vi "GetPositionDegreesPosition.vi"(0 "StepMotor in":refnum<class "StepMotor.lvclass">, 2 "Редукция":dbl, 3 "Разрешение энкодера":dbl, 5 "error in (no error)":errorcluster) -> (14 "StepMotor out":refnum<class "StepMotor.lvclass">, 16 "Значение":dbl, 17 "+360 -360":bool, 18 "+ 0 -":bool, 19 "error out":errorcluster)   [LabVIEW 2010, in "StepMotor.lvclass"]
uses:
  StepMotor.lvclass
panel:
  out "BadValue":bool
  out "RawValue":dbl
  out "МножПриведШкалы360":dbl
  out "КолИмпулОборот":dbl
  out "Текущая позиция":dbl
  out "Предыдущая позиция":dbl
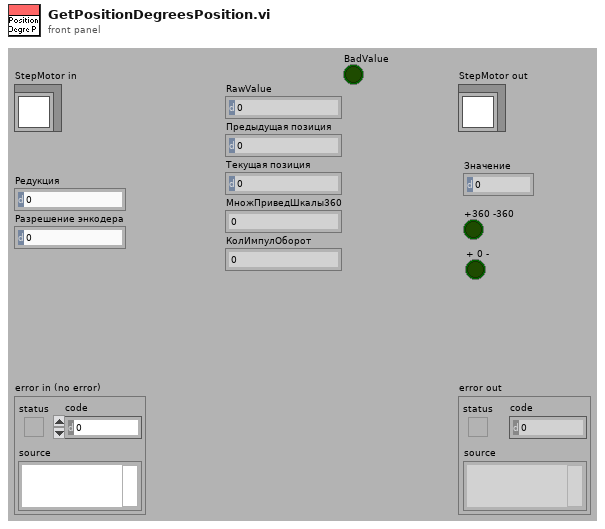
[diagram p1: front panel]
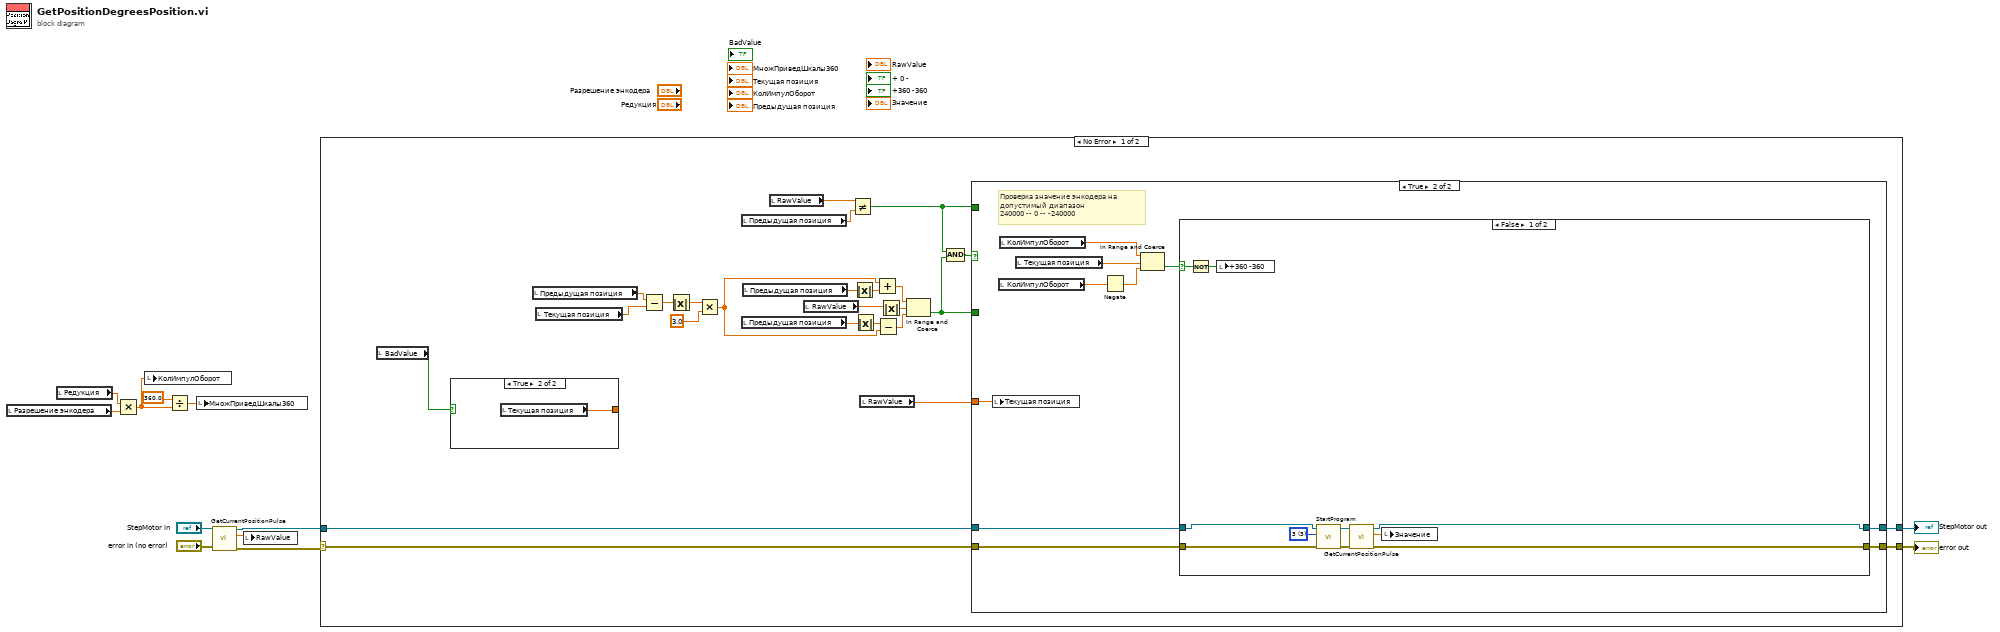
[diagram p0: block diagram]
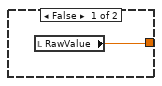
[diagram p2: hidden frame]
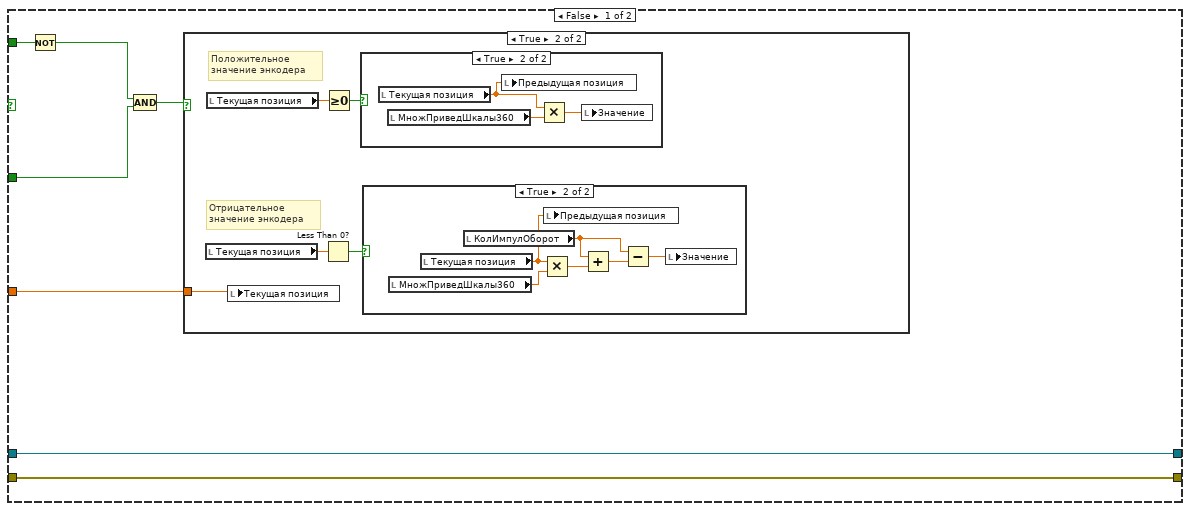
[diagram p3: hidden frame]
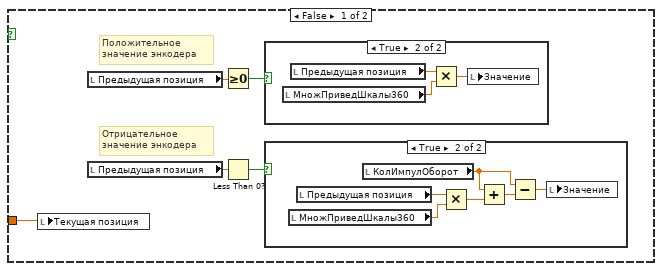
[diagram p4: hidden frame]
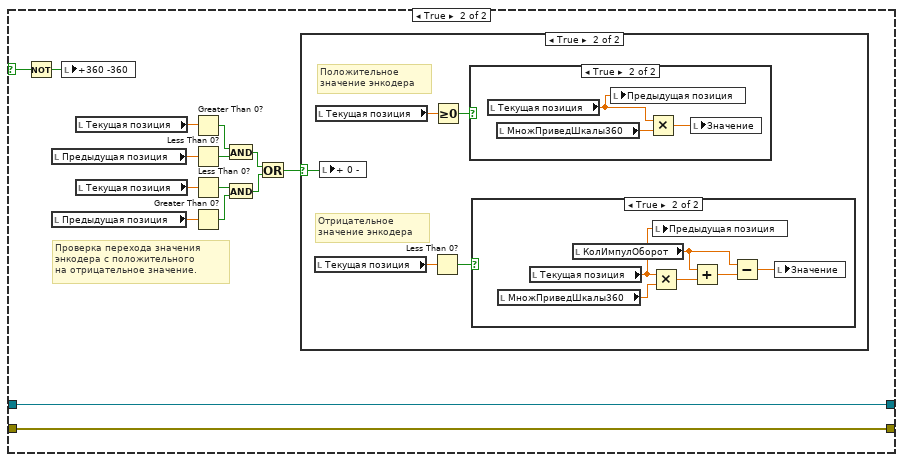
[diagram p9: hidden frame]
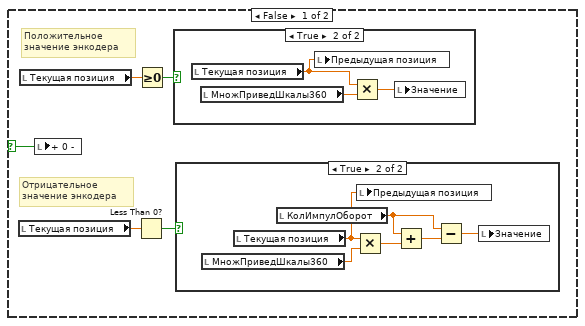
[diagram p10: hidden frame]
diagram:
  n1 = local read "Разрешение энкодера"() -> (w7:dbl)
  n2 = local read "Редукция"() -> (w6:dbl)
  n3 = Multiply(x=w6, y=w7) -> (x*y=w9:dbl)
  n4 = local write "КолИмпулОборот"(w9) -> ()
  n5 = Divide(x=360.0, y=w9) -> (x/y=w10:dbl)
  n6 = local write "МножПриведШкалы360"(w10) -> ()
  n7 = call-dynamic "GetCurrentPositionPulse.vi"("error in (no error)"="error in (no error)", "StepMotor in"="StepMotor in") -> ("error out"=w1:errorcluster, "Текущая позиция"=w5:dbl, "StepMotor out"=w2:refnum<class "StepMotor.lvclass">)  [unwired: 7 in]
  n8 = local write "RawValue"(w5) -> ()
  n9 = case shown="No Error" w1 {
    selector: w1 -> [w18 w138]
    tunnel: w2 -> [w19 w139]
    tunnel: [w37 w139] -> w11
    tunnel: [w36 w138] -> w12
    frame No Error {
      n10 = local read "BadValue"() -> (w16:bool)
      n11 = case shown="True" w16 {
        tunnel: [w38 w39] -> _
        frame False {
          n12 = local read "RawValue"() -> (w38:dbl)
        }
        frame True {
          n13 = local read "Текущая позиция"() -> (w39:dbl)
        }
      }
      n14 = local read "Предыдущая позиция"() -> (w24:dbl)
      n15 = local read "Текущая позиция"() -> (w13:dbl)
      n16 = Subtract(x=w24, y=w13) -> (x-y=w23:dbl)
      n17 = Absolute Value(x=w23) -> (abs(x)=w21:dbl)
      n18 = Multiply(x=w21, y=3.0) -> (x*y=w22:dbl)
      n19 = local read "Предыдущая позиция"() -> (w35:dbl)
      n20 = local read "Предыдущая позиция"() -> (w28:dbl)
      n21 = local read "Предыдущая позиция"() -> (w25:dbl)
      n22 = local read "RawValue"() -> (w15:dbl)
      n23 = local read "RawValue"() -> (w17:dbl)
      n24 = Not Equal?(x=w15, y=w35) -> (x != y?=w32:bool)
      n25 = Absolute Value(x=w25) -> (abs(x)=w29:dbl)
      n26 = Absolute Value(x=w28) -> (abs(x)=w27:dbl)
      n27 = local read "RawValue"() -> (w14:dbl)
      n28 = Add(x=w22, y=w29) -> (x+y=w30:dbl)
      n29 = Subtract(x=w27, y=w22) -> (x-y=w26:dbl)
      n30 = Absolute Value(x=w17) -> (abs(x)=w31:dbl)
      n31 = In Range and Coerce(upper limit=w30, x=w31, lower limit=w26) -> (In Range?=w33:bool)  [unwired: 1 out]
      n32 = Compound Arithmetic op=AND(w32, w33) -> (w34:bool)
      n33 = case shown="True" w34 {
        tunnel: w33 -> [w41 _]
        tunnel: w32 -> [w44 _]
        tunnel: w19 -> [w46 w84]
        tunnel: w18 -> [w45 w83]
        tunnel: [w46 w82] -> w37
        tunnel: [w45 w81] -> w36
        tunnel: w14 -> [w40 w75]
        frame False {
          n34 = Not(x=w44) -> (.not. x?=w43:bool)
          n35 = Compound Arithmetic op=AND(w43, w41) -> (w42:bool)
          n36 = case shown="True" w42 {
            tunnel: w40 -> [w47 w61]
            frame False {
              # "Отрицательное \nзначение энкодера"
              # "Положительное \nзначение энкодера"
              n37 = local write "Текущая позиция"(w47) -> ()
              n38 = local read "Предыдущая позиция"() -> (w49:dbl)
              n39 = local read "Предыдущая позиция"() -> (w48:dbl)
              n40 = Greater Or Equal To 0?(x=w49) -> (x >= 0?=w51:bool)
              n41 = Less Than 0?(x=w48) -> (x < 0?=w50:bool)
              n42 = case shown="True" w51 {
                frame False {
                }
                frame True {
                  n43 = local read "МножПриведШкалы360"() -> (w60:dbl)
                  n44 = local read "Предыдущая позиция"() -> (w58:dbl)
                  n45 = Multiply(x=w58, y=w60) -> (x*y=w59:dbl)
                  n46 = local write "Значение"(w59) -> ()
                }
              }
              n47 = case shown="True" w50 {
                frame False {
                }
                frame True {
                  n48 = local read "МножПриведШкалы360"() -> (w57:dbl)
                  n49 = local read "Предыдущая позиция"() -> (w56:dbl)
                  n50 = local read "КолИмпулОборот"() -> (w54:dbl)
                  n51 = Multiply(x=w56, y=w57) -> (x*y=w55:dbl)
                  n52 = Add(x=w54, y=w55) -> (x+y=w53:dbl)
                  n53 = Subtract(x=w54, y=w53) -> (x-y=w52:dbl)
                  n54 = local write "Значение"(w52) -> ()
                }
              }
            }
            frame True {
              # "Отрицательное \nзначение энкодера"
              # "Положительное \nзначение энкодера"
              n55 = local read "Текущая позиция"() -> (w65:dbl)
              n56 = local read "Текущая позиция"() -> (w64:dbl)
              n57 = local write "Текущая позиция"(w61) -> ()
              n58 = Less Than 0?(x=w65) -> (x < 0?=w62:bool)
              n59 = Greater Or Equal To 0?(x=w64) -> (x >= 0?=w63:bool)
              n60 = case shown="True" w63 {
                frame False {
                }
                frame True {
                  n61 = local read "Текущая позиция"() -> (w72:dbl)
                  n62 = local read "МножПриведШкалы360"() -> (w74:dbl)
                  n63 = local write "Предыдущая позиция"(w72) -> ()
                  n64 = Multiply(x=w72, y=w74) -> (x*y=w73:dbl)
                  n65 = local write "Значение"(w73) -> ()
                }
              }
              n66 = case shown="True" w62 {
                frame False {
                }
                frame True {
                  n67 = local read "МножПриведШкалы360"() -> (w71:dbl)
                  n68 = local read "Текущая позиция"() -> (w70:dbl)
                  n69 = local read "КолИмпулОборот"() -> (w68:dbl)
                  n70 = Multiply(x=w70, y=w71) -> (x*y=w69:dbl)
                  n71 = local write "Предыдущая позиция"(w70) -> ()
                  n72 = Add(x=w68, y=w69) -> (x+y=w67:dbl)
                  n73 = Subtract(x=w68, y=w67) -> (x-y=w66:dbl)
                  n74 = local write "Значение"(w66) -> ()
                }
              }
            }
          }
        }
        frame True {
          # "Проверка значение энкодера на\nдопустимый диапазон \n240000 -- 0 -- -240000"
          n75 = local write "Текущая позиция"(w75) -> ()
          n76 = local read "КолИмпулОборот"() -> (w77:dbl)
          n77 = local read "КолИмпулОборот"() -> (w78:dbl)
          n78 = local read "Текущая позиция"() -> (w76:dbl)
          n79 = Negate(x=w77) -> (-x=w80:dbl)
          n80 = In Range and Coerce(upper limit=w78, x=w76, lower limit=w80) -> (In Range?=w79:bool)  [unwired: 1 out]
          n81 = case shown="False" w79 {
            selector: w79 -> [w91 w95]
            tunnel: w84 -> [w88 w98]
            tunnel: w83 -> [w87 w97]
            tunnel: [w93 w98] -> w82
            tunnel: [w92 w97] -> w81
            frame False {
              w94 = u16 3 items=["0", "1", "2", "3", "4", "5", "6", "7"] ("Номер банка программ")
              n82 = Not(x=w91) -> (.not. x?=w90:bool)
              n83 = local write "+360 -360"(w90) -> ()
              n84 = call-dynamic "StartProgram.vi"("error in (no error)"=w87, "Номер банка программ"=w94, "StepMotor in"=w88) -> ("error out"=w85:errorcluster, "StepMotor out"=w86:refnum<class "StepMotor.lvclass">)  [unwired: 7 in]
              n85 = call-dynamic "GetCurrentPositionPulse.vi"("error in (no error)"=w85, "StepMotor in"=w86) -> ("error out"=w92:errorcluster, "Текущая позиция"=w89:dbl, "StepMotor out"=w93:refnum<class "StepMotor.lvclass">)  [unwired: 7 in]
              n86 = local write "Значение"(w89) -> ()
            }
            frame True {
              # "Проверка перехода значения \nэнкодера с положительного\nна отрицательное значение."
              n87 = Not(x=w95) -> (.not. x?=w96:bool)
              n88 = local read "Предыдущая позиция"() -> (w100:dbl)
              n89 = local read "Предыдущая позиция"() -> (w99:dbl)
              n90 = local write "+360 -360"(w96) -> ()
              n91 = local read "Текущая позиция"() -> (w102:dbl)
              n92 = local read "Текущая позиция"() -> (w101:dbl)
              n93 = Greater Than 0?(x=w102) -> (x > 0?=w105:bool)
              n94 = Less Than 0?(x=w100) -> (x < 0?=w106:bool)
              n95 = Less Than 0?(x=w101) -> (x < 0?=w104:bool)
              n96 = Greater Than 0?(x=w99) -> (x > 0?=w103:bool)
              n97 = And(x=w105, y=w106) -> (x .and. y?=w107:bool)
              n98 = And(x=w104, y=w103) -> (x .and. y?=w108:bool)
              n99 = Or(x=w107, y=w108) -> (x .or. y?=w109:bool)
              n100 = case shown="True" w109 {
                selector: w109 -> [w110 w124]
                frame False {
                  # "Отрицательное \nзначение энкодера"
                  # "Положительное \nзначение энкодера"
                  n101 = local read "Текущая позиция"() -> (w114:dbl)
                  n102 = local read "Текущая позиция"() -> (w113:dbl)
                  n103 = local write "+ 0 -"(w110) -> ()
                  n104 = Less Than 0?(x=w114) -> (x < 0?=w111:bool)
                  n105 = Greater Or Equal To 0?(x=w113) -> (x >= 0?=w112:bool)
                  n106 = case shown="True" w112 {
                    frame False {
                    }
                    frame True {
                      n107 = local read "Текущая позиция"() -> (w121:dbl)
                      n108 = local read "МножПриведШкалы360"() -> (w123:dbl)
                      n109 = local write "Предыдущая позиция"(w121) -> ()
                      n110 = Multiply(x=w121, y=w123) -> (x*y=w122:dbl)
                      n111 = local write "Значение"(w122) -> ()
                    }
                  }
                  n112 = case shown="True" w111 {
                    frame False {
                    }
                    frame True {
                      n113 = local read "МножПриведШкалы360"() -> (w120:dbl)
                      n114 = local read "Текущая позиция"() -> (w119:dbl)
                      n115 = local read "КолИмпулОборот"() -> (w117:dbl)
                      n116 = Multiply(x=w119, y=w120) -> (x*y=w118:dbl)
                      n117 = local write "Предыдущая позиция"(w119) -> ()
                      n118 = Add(x=w117, y=w118) -> (x+y=w116:dbl)
                      n119 = Subtract(x=w117, y=w116) -> (x-y=w115:dbl)
                      n120 = local write "Значение"(w115) -> ()
                    }
                  }
                }
                frame True {
                  # "Отрицательное \nзначение энкодера"
                  # "Положительное \nзначение энкодера"
                  n121 = local read "Текущая позиция"() -> (w128:dbl)
                  n122 = local read "Текущая позиция"() -> (w127:dbl)
                  n123 = local write "+ 0 -"(w124) -> ()
                  n124 = Less Than 0?(x=w128) -> (x < 0?=w125:bool)
                  n125 = Greater Or Equal To 0?(x=w127) -> (x >= 0?=w126:bool)
                  n126 = case shown="True" w126 {
                    frame False {
                    }
                    frame True {
                      n127 = local read "Текущая позиция"() -> (w135:dbl)
                      n128 = local read "МножПриведШкалы360"() -> (w137:dbl)
                      n129 = local write "Предыдущая позиция"(w135) -> ()
                      n130 = Multiply(x=w135, y=w137) -> (x*y=w136:dbl)
                      n131 = local write "Значение"(w136) -> ()
                    }
                  }
                  n132 = case shown="True" w125 {
                    frame False {
                    }
                    frame True {
                      n133 = local read "МножПриведШкалы360"() -> (w134:dbl)
                      n134 = local read "Текущая позиция"() -> (w133:dbl)
                      n135 = local read "КолИмпулОборот"() -> (w131:dbl)
                      n136 = Multiply(x=w133, y=w134) -> (x*y=w132:dbl)
                      n137 = local write "Предыдущая позиция"(w133) -> ()
                      n138 = Add(x=w131, y=w132) -> (x+y=w130:dbl)
                      n139 = Subtract(x=w131, y=w130) -> (x-y=w129:dbl)
                      n140 = local write "Значение"(w129) -> ()
                    }
                  }
                }
              }
            }
          }
        }
      }
    }
    frame Error {
    }
  }
  "error out" <- w12
  "StepMotor out" <- w11
